vi "Sound Spectrogram Advanced.vi"() -> ()   [LabVIEW 2021]
doc: "This VI illustrates how to perform simultaneous sound IO, i.e., how to continuously play the sound acquired from a microphone. It requires the use of a microphone attached to the sound card. You can specify the IDs of the input and output devices, the frequency to sample at, and the buffer size for both devices. Higher frequencies have better quality, but demand more resources and are limited by the capabilities of your sound card. A large number of samples decreases the risk of glitches, but increases the delay between acquisition and playback."
uses:
  <vilib>/Analysis/4window.llb/windowTd.ctl
  SubVI/Spectrogram States.ctl
  SubVI/Global Variable Operation.ctl
  <vilib>/sound2/lvsound2.llb/Sampling Mode.ctl
  <vilib>/measure/maspectr.llb/Power Spectrum and PSD Export Mode.ctl
  <vilib>/sound2/lvsound2.llb/Sound Input Task ID.ctl
  <vilib>/sound2/lvsound2.llb/Sound Input Read (DBL).vi
  <vilib>/measure/maspectr.llb/FFT Power Spectrum and PSD for N Chan.vi
  <vilib>/measure/NI_MAPro.lvlib
  <vilib>/Analysis/NI_AALPro.lvlib
panel:
  in  "Stop":bool
  in  "Tab Control":enum32{"Signal", "Settings"}(tab)
  in  "Frequency\n[Hz]":cluster{dbl, dbl}(slide)={0.0, 3000.0} scale=0.0..4000.0
  in  "Intensity\n[dB]":cluster{dbl, dbl}(slide)={-120.0, -20.0}
  out "Sound Spectrogram":dbl[][](graph)
  out "Acquired Sound":waveform(dbl)[](graph)
  out "Power Spectral Density":cluster{"f0":dbl, "df":dbl, "magnitude":dbl[]}[](graph)
  in  "Sampling":T1={"Rate [S/s]"=44100.0, "Channels"=2.0, "Resolution [Bits]"=16.0} {"Rate [S/s]" format="%#_6p"}
  in  "Interval [s]":dbl=0.1 min=0.1 max=5.0 step=0.1
  in  "Window":T2=1 items=["Rectangle"=0, "Hanning"=1, "Hamming"=2, "Blackman-Harris"=3, "Exact Blackman"=4, "Blackman"=5, "Flat Top"=6, "4 Term B-Harris "=7, "7 Term B-Harris"=8, "Low Sidelobe"=9, "Blackman Nuttall"=11, "Triangle"=30, "Bartlett-Hanning"=31, "Bohman"=32, "Parzen"=33, "Welch"=34, "Kaiser"=60, "Dolph-Chebyshev"=61, "Gaussian"=62]
  in  "Sound Input Device ID":u32
  # "Sound Signal and Frequency Spectrum"
  # "Record sound from the computer input device.\nShow recorded signal and its power spectrum."
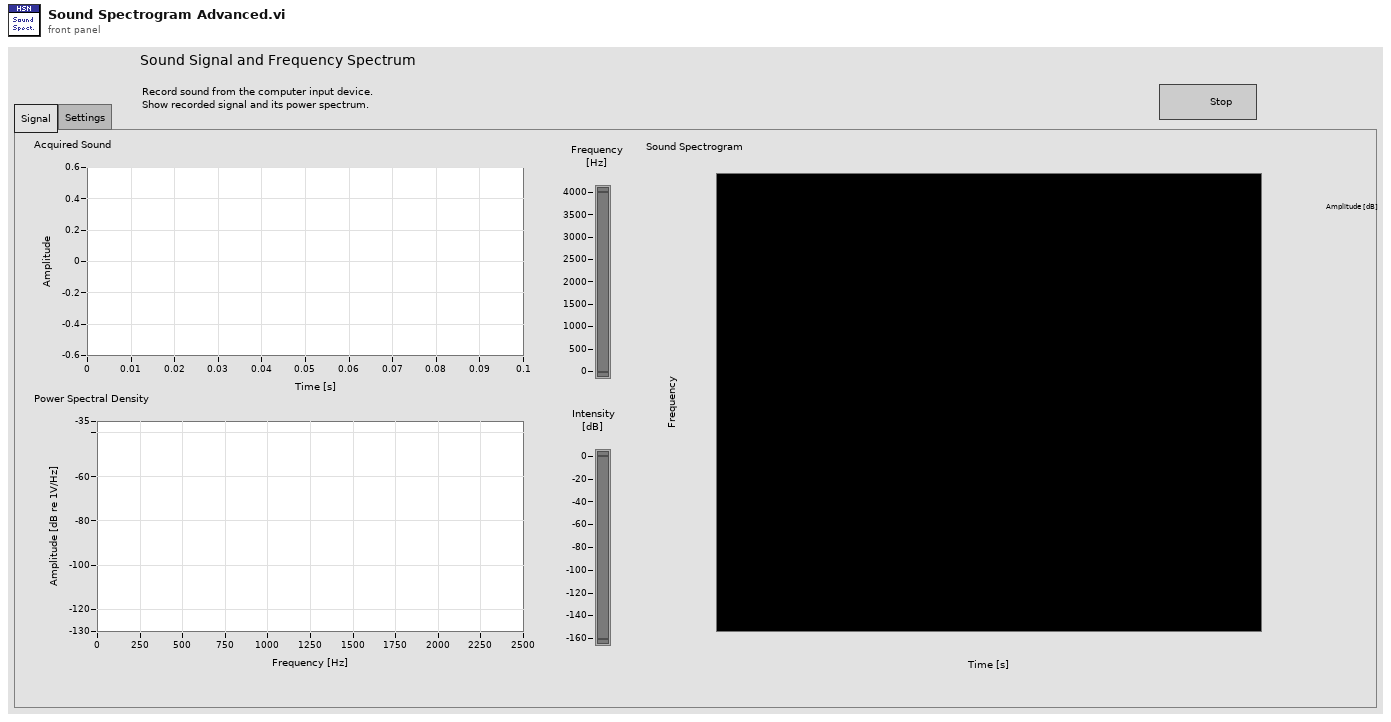
[diagram p1: front panel]
types:
  T1 = cluster{"Rate [S/s]":dbl, "Channels":dbl, "Resolution [Bits]":dbl}
  T2 = typedef "NI_AALPro.lvlib/windowTd.ctl" = u32
  T3 = typedef "Global Variable Operation.ctl" = enum16{"Clear", "Set", "Get"}
  T4 = typedef "Spectrogram States.ctl" = enum16{"Initialize", "Idle", "Acquire", "Process", "Display", "Rescale", "Shutdown", "Quit"}
  T5 = typedef "Sound Input Task ID.ctl" = u32
  T6 = typedef "Sampling Mode.ctl" = i32
  T7 = typedef "NI_MAPro.lvlib/Power Spectrum and PSD Export Mode.ctl" = u16
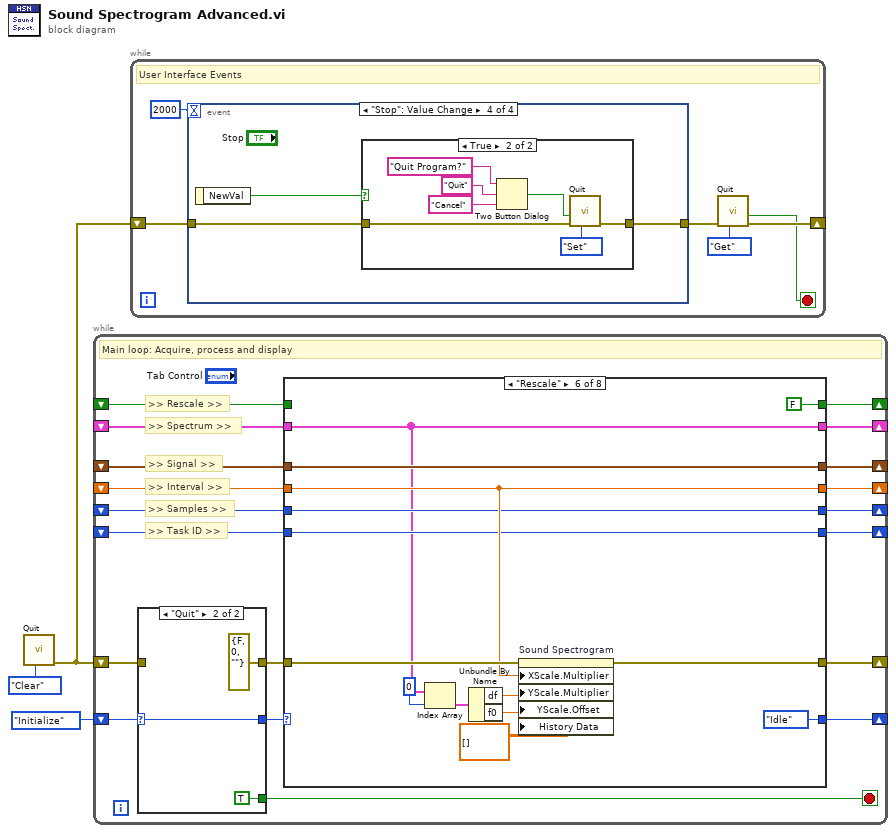
[diagram p0: block diagram]
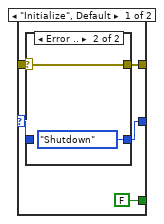
[diagram p2: hidden frame]
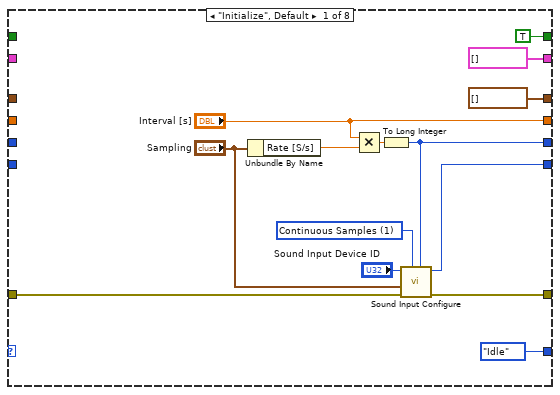
[diagram p4: hidden frame]
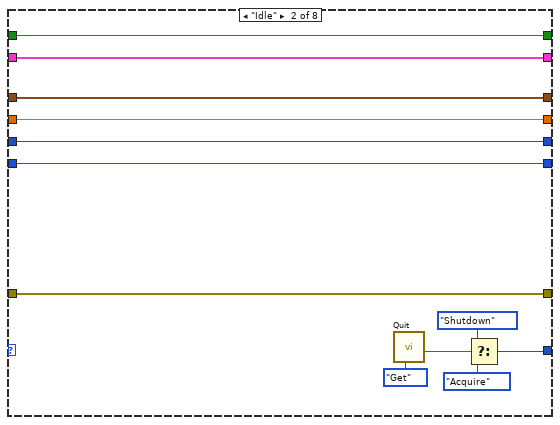
[diagram p5: hidden frame]
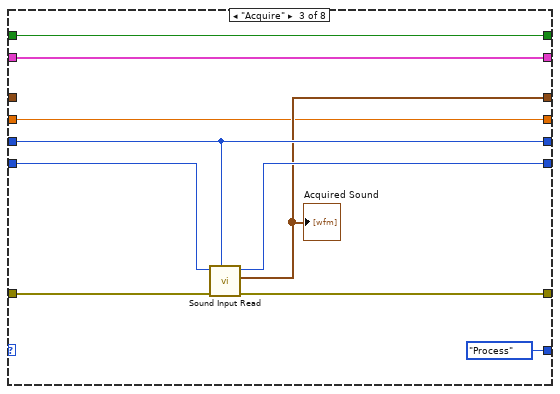
[diagram p6: hidden frame]
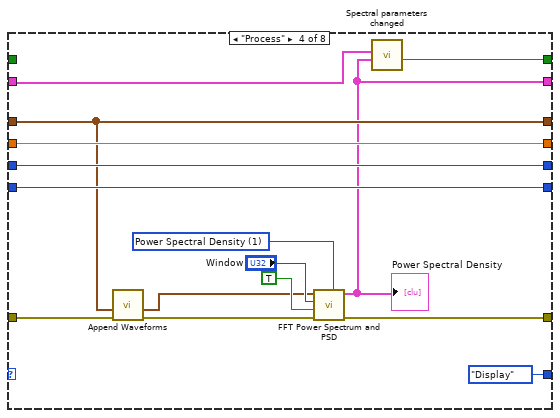
[diagram p7: hidden frame]
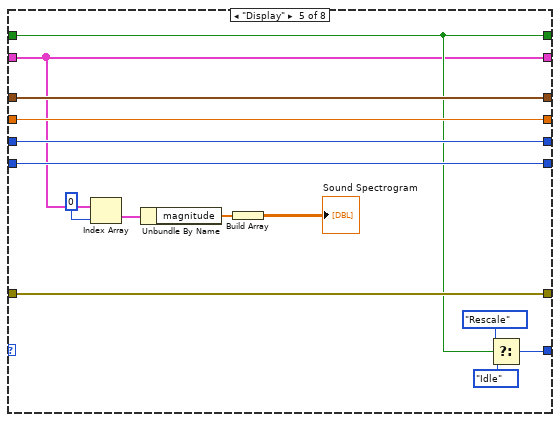
[diagram p8: hidden frame]
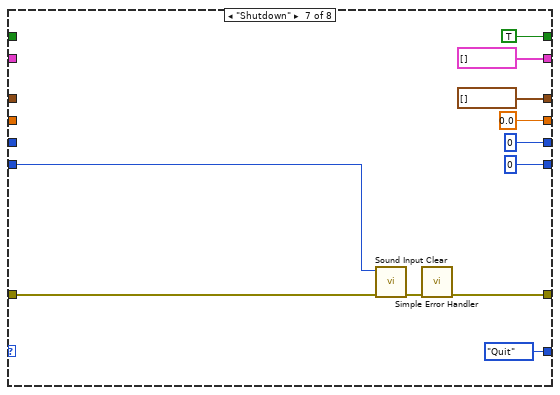
[diagram p9: hidden frame]
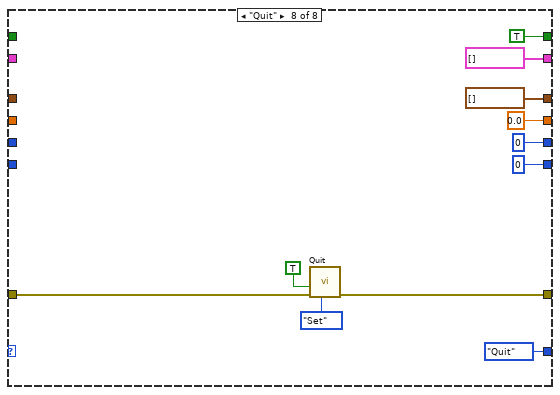
[diagram p10: hidden frame]
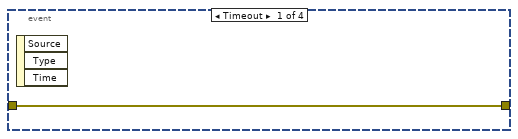
[diagram p11: hidden frame]
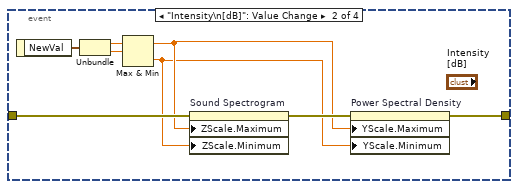
[diagram p12: hidden frame]
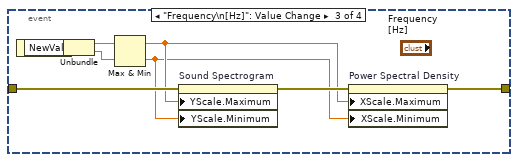
[diagram p13: hidden frame]
diagram:
  n1 = call "Quit.vi"("Operation"=Global_Variable_Operation."Clear") -> ("Error Out"=w1:errorcluster)  [unwired: 9 in, 1 out]
  n2 = while {
    shift-right: [w22] -> _
    shift-left: w1 -> [w8]
    shift-right: [w21] -> _
    shift-left: _ -> [w20]
    shift-right: [w19] -> _
    shift-left: _ -> [w18]
    shift-right: [w17] -> _
    shift-left: Spectrogram_States."Initialize" ("State") -> [w5]
    shift-right: [w16] -> _
    shift-left: _ -> [w15]
    shift-right: [w14] -> _
    shift-left: _ -> [w13]
    shift-right: [w12] -> _
    shift-left: _ -> [w11]
    shift-right: [w10] -> _
    shift-left: _ -> [w9]
    stop <- w4 stop-if-true
    # ">> Spectrum >>"
    # ">> Rescale >>"
    # ">> Interval >>"
    # ">> Signal >>"
    # ">> Task ID >>"
    # ">> Samples >>"
    # "Main loop: Acquire, process and display"
    n3 = case shown="\"Quit\"" w5 {
      selector: w5 -> [w24 w34]
      tunnel: w8 -> [w27 _]
      tunnel: [w26 errorcluster {"status"=FALSE, "code"=0, "source"=""} ("error IO")] -> w7
      tunnel: [w25 w34] -> w6
      tunnel: [FALSE TRUE] -> w4
      frame "Initialize", Default {
        n4 = case shown="Error .." w27 {
          selector: w27 -> [w29 w31]
          tunnel: [w29 w31] -> w26
          tunnel: w24 -> [w28 _]
          tunnel: [w28 Spectrogram_States."Shutdown" ("State")] -> w25
          frame No Error {
          }
          frame Error {
          }
        }
      }
      frame "Quit" {
      }
    }
    n5 = case shown="\"Rescale\"" w6 {
      tunnel: [w43 w51 w66 w82 w95 w104 w122 w126] -> w22
      tunnel: w7 -> [w42 w51 w67 w76 w95 w112 w124 w127]
      tunnel: [w41 w60 w68 w80 w99 w108 0 0] -> w21
      tunnel: w20 -> [_ w60 w68 w80 w99 w108 _ _]
      tunnel: [w40 w59 w69 w81 w98 w107 T5 0 ("task ID out") T5 0 ("task ID out")] -> w19
      tunnel: w18 -> [_ w59 w70 w81 w98 w107 w120 _]
      tunnel: [Spectrogram_States."Idle" ("State") w56 Spectrogram_States."Process" ("State") Spectrogram_States."Display" ("State") w91 Spectrogram_States."Idle" ("State") Spectrogram_States."Quit" ("State") Spectrogram_States."Quit" ("State")] -> w17
      tunnel: [waveform(dbl)[] [] ("data") w55 w64 w74 w97 w106 waveform(dbl)[] [] ("data") waveform(dbl)[] [] ("data")] -> w16
      tunnel: w15 -> [_ w55 _ w74 w97 w106 _ _]
      tunnel: [cluster{"f0":dbl, "df":dbl, "magnitude":dbl[]}[] [] ("Power Spectrum / PSD") w54 w63 w73 w88 w105 cluster{"f0":dbl, "df":dbl, "magnitude":dbl[]}[] [] ("Power Spectrum / PSD") cluster{"f0":dbl, "df":dbl, "magnitude":dbl[]}[] [] ("Power Spectrum / PSD")] -> w14
      tunnel: w13 -> [_ w54 w63 w72 w88 w105 _ _]
      tunnel: ["Interval [s]" w53 w62 w78 w96 w109 0.0 ("Block Size [s]") 0.0 ("Block Size [s]")] -> w12
      tunnel: w11 -> [_ w53 w62 w78 w96 w109 _ _]
      tunnel: [TRUE w52 w61 w71 w94 FALSE TRUE TRUE] -> w10
      tunnel: w9 -> [_ w52 w61 _ w94 _ _ _]
      frame "Initialize", Default {
        w45 = T6 1 items=["Finite Samples", "Continuous Samples"] ("sample mode")
        n6 = Unbundle By Name("Sampling") -> ("Rate [S/s]"=w47:dbl)
        n7 = Multiply(x="Interval [s]", y=w47) -> (x*y=w48:dbl)
        n8 = To Long Integer(number=w48) -> (32bit integer=w41:i32)
        n9 = call <vilib>:"Sound Input Configure.vi"("number of samples/ch"=w41, "sample mode"=w45, "error in (no error)"=w42, "sound format"="Sampling", "device ID"="Sound Input Device ID") -> ("error out"=w43:errorcluster, "task ID"=w40:T5)  [unwired: 5 in]
      }
      frame "Idle" {
        n10 = call "Quit.vi"("Operation"=Global_Variable_Operation."Get") -> ("Quit?"=w50:bool)  [unwired: 9 in, 1 out]
        n11 = Select(t=Spectrogram_States."Shutdown" ("State"), s=w50, f=Spectrogram_States."Acquire" ("State")) -> (s? t:f=w56:T4)
      }
      frame "Acquire" {
        n12 = call-poly <vilib>:"Sound Input Read.vi"("number of samples/ch"=w68, "error in (no error)"=w67, "task ID"=w70) -> ("error out"=w66:errorcluster, "data"=w64:waveform(dbl)[], "task ID out"=w69:T5)  [unwired: 6 in]
        "Acquired Sound" <- w64
      }
      frame "Process" {
        w85 = T7 1 items=["Power Spectrum", "Power Spectral Density"] ("export mode")
        n13 = call "Append Waveforms.vi"("Error In"=w76, "Signals In"=w74) -> ("Error Out"=w75:errorcluster, "Appended Signals Out"=w77:waveform(dbl)[])  [unwired: 8 in]
        n14 = call-poly <vilib>:"FFT Power Spectrum and PSD.vi"("export mode"=w85, "error in (no error)"=w75, "dB On (F)"=TRUE, "window"="Window", "time signals"=w77) -> ("error out"=w82:errorcluster, "Power Spectrum / PSD"=w73:cluster{"f0":dbl, "df":dbl, "magnitude":dbl[]}[])  [unwired: 3 in, 2 out]
        "Power Spectral Density" <- w73
        n15 = call "Spectral parameters changed.vi"("Old PSDs"=w73, "New PSDs"=w72) -> ("Spectral parameters changed"=w71:bool)  [unwired: 9 in]
      }
      frame "Display" {
        n16 = Index Array(array=w88, index=0 ("index (row)")) -> (element=w87:cluster{"f0":dbl, "df":dbl, "magnitude":dbl[]})
        n17 = Unbundle By Name(w87) -> ("magnitude"=w86:dbl[])
        n18 = Build Array(w86) -> (→"Sound Spectrogram":dbl[][])
        n19 = Select(t=Spectrogram_States."Rescale" ("State"), s=w94, f=Spectrogram_States."Idle" ("State")) -> (s? t:f=w91:T4)
      }
      frame "Rescale" {
        n20 = Index Array(array=w105, index=0) -> (element=w113:cluster{"f0":dbl, "df":dbl, "magnitude":dbl[]})
        n21 = Unbundle By Name(w113) -> ("df"=w110:dbl, "f0"=w111:dbl)
        n22 = property on="Sound Spectrogram" class="IntChart (strict)"(error in=w112, "XScale.Multiplier"=w109, "YScale.Multiplier"=w110, "YScale.Offset"=w111, "History Data"=dbl[][] []) -> (error out=w104:errorcluster)  [unwired: 1 in, 1 out]
      }
      frame "Shutdown" {
        n23 = call <vilib>:"Sound Input Clear.vi"("error in (no error)"=w124, "task ID"=w120) -> ("error out"=w123:errorcluster)  [unwired: 9 in]
        n24 = call <vilib>:"Simple Error Handler.vi"("error in (no error)"=w123) -> ("error out"=w122:errorcluster)  [unwired: 4 in, 4 out]
      }
      frame "Quit" {
        n25 = call "Quit.vi"("Operation"=Global_Variable_Operation."Set", "Error In"=w127, "Quit"=TRUE) -> ("Error Out"=w126:errorcluster)  [unwired: 7 in, 1 out]
      }
    }
  }
  n26 = while {
    shift-right: [w139] -> _
    shift-left: w1 -> [w141]
    stop <- w137 stop-if-true
    # "User Interface Events"
    n27 = event shown="[3] \"Stop\": Value Change" {
      selector: _ -> [_ _ _ _]
      dyn-events: _ -> [_ _ _ _]
      timeout: 2000 -> [_ _ _ _]
      tunnel: [w142 w145 w155 w159] -> w140
      tunnel: w141 -> [w142 w150 w153 w160]
      event Timeout {
        n28 = event-data() -> ()  [unwired: 1 in, 3 out]
      }
      event "Intensity\n[dB]": Value Change {
        n29 = event-data() -> ("NewVal"=w147:cluster{dbl, dbl})  [unwired: 1 in]
        n30 = Unbundle(w147) -> (w149:dbl, w148:dbl)
        n31 = Max & Min(x=w149, y=w148) -> (max(x,y)=w144:dbl, min(x,y)=w143:dbl)
        n32 = property on="Sound Spectrogram" class="IntChart (strict)"(error in=w150, "ZScale.Maximum"=w144, "ZScale.Minimum"=w143) -> (error out=w146:errorcluster)  [unwired: 1 in, 1 out]
        n33 = property on="Power Spectral Density" class="WFGraph (strict)"(error in=w146, "YScale.Maximum"=w144, "YScale.Minimum"=w143) -> (error out=w145:errorcluster)  [unwired: 1 in, 1 out]
      }
      event "Frequency\n[Hz]": Value Change {
        n34 = event-data() -> ("NewVal"=w156:cluster{dbl, dbl})  [unwired: 1 in]
        n35 = Unbundle(w156) -> (w158:dbl, w157:dbl)
        n36 = Max & Min(x=w158, y=w157) -> (max(x,y)=w152:dbl, min(x,y)=w151:dbl)
        n37 = property on="Sound Spectrogram" class="IntChart (strict)"(error in=w153, "YScale.Maximum"=w152, "YScale.Minimum"=w151) -> (error out=w154:errorcluster)  [unwired: 1 in, 1 out]
        n38 = property on="Power Spectral Density" class="WFGraph (strict)"(error in=w154, "XScale.Maximum"=w152, "XScale.Minimum"=w151) -> (error out=w155:errorcluster)  [unwired: 1 in, 1 out]
      }
      event "Stop": Value Change {
        n39 = event-data() -> ("NewVal"=w161:bool)  [unwired: 1 in]
        n40 = case shown="True" w161 {
          tunnel: w160 -> [w162 w165]
          tunnel: [w162 w164] -> w159
          frame False {
          }
          frame True {
            n41 = Two Button Dialog(message="Quit Program?" ("Quit Program?"), 1:"Cancel" ("F button name (\"Cancel\")"), 2:"Quit" ("T button name (\"OK\")")) -> (T button?=w166:bool)
            n42 = call "Quit.vi"("Operation"=Global_Variable_Operation."Set", "Error In"=w165, "Quit"=w166) -> ("Error Out"=w164:errorcluster)  [unwired: 7 in, 1 out]
          }
        }
      }
    }
    n43 = call "Quit.vi"("Operation"=Global_Variable_Operation."Get", "Error In"=w140) -> ("Error Out"=w139:errorcluster, "Quit?"=w137:bool)  [unwired: 8 in]
  }
